vi "ADC SNR_new_beforeChn.vi"(8 "error in (no error)":errorcluster, 9 "Sequence parameters":string[][](array[string])=[["Min limit", "Max limit", "Register sheet file", "Register Sheet"], ["", "", "CC2600.xls", "TX_BLE;Trim"], ["Reg write (addr;value)", "Operating frequency [Hz]", "", ""], ["NA", "2.44G", "", ""]], 10 "Run type":i32, 11 "Method parameters":T4={"Dev"={"Do not disturb DUT"=FALSE, "XOSC"=32000000.0, "Board type"="", "EM"="", "Configure tempboard"=TRUE, "Device specific info"=[], "Generic Object"=refnum}, "Method"={"Run type"=1, "Test name"="Current LPM2 4", "Comment"="", "Results folder"="", "AFC"=enum."Off", "Method name"="Current LPM2 4", "Method results"={"Excel brief report"=FALSE, "Spotfire report"=FALSE, "Starfish report"=FALSE}, "Operator"="", "Reference time"=timestamp(0 s since 1904-01-01), "AFC delay"=0.0, "Initialization"=enum."Enabled", "MD5 Sum"="", "HW addon board"=enum."None", "AFC Regsheet"="", "AFC Regfile"=path "", "dummy"=0.0}, "Inst"={"Instr"={"PS1"={"Name"="", "GPIB address"="", "VISA session"=""}, "PS2"={"Name"="", "GPIB address"="", "VISA session"=""}, "TC1"={"Name"="", "GPIB address"="", "VISA session"=""}, "TC2"={"Name"="", "GPIB address"="", "VISA session"=""}, "SA1"={"Name"="", "GPIB address"="", "VISA session"=""}, "SA2"={"Name"="", "GPIB address"="", "VISA session"=""}, "SG1"={"Name"="", "GPIB address"="", "VISA session"=""}, "SG2"={"Name"="", "GPIB address"="", "VISA session"=""}, "SG3"={"Name"="", "GPIB address"="", "VISA session"=""}, "MI1"={"Name"="", "GPIB address"="", "VISA session"=""}, "MI2"={"Name"="", "GPIB address"="", "VISA session"=""}, "SW SA"={"Name"="", "Controller addr"=""}, "SW SG"={"Name"="", "Controller addr"=""}, "MI3"={"Name"="", "GPIB address"="", "VISA session"=""}}, "Switchbox"={"RF Path"=0, "Cal compensation"=enum."TX", "Switchbox gain mode"="", "State"=enum."TX"}, "Instr to control (i.e. SA1)"="Default", "Intrument info string"=""}, "Sequence parameters"=[["Weight", "Min Limit", "Max Limit", "Register Sheet", "", "", "", "", "", "", "", "", ""], ["Vital", "", "1", "LPM2", "", "", "", "", "", "", "", "", ""], ["Resolution", "Reg write (addr;value)", "Chip mode", "Range", "", "", "", "", "", "", "", "", ""], ["u", "NA", "", "auto", "", "", "", "", "", "", "", "", ""]], "Cond"={"Temp logged"=25.0, "VDD1_PS1_6V"=-999.0, "VDD2_PS1_25V"=-999.0, "VDD4_PS2_25V"=-999.0, "VDD3_PS2_6V"=-999.0}, "Meas config"={"X-axis inner loop index"=32000000, "Y-axis outer loop index"=32000000, "X-axis"=[], "Y-axis"=[], "X-axis array req size"=32000000, "Y-axis array req size"=32000000, "Param description"=[], "Use meas clust for reporting"=FALSE, "Parameter index (page)"=0, "X-axis name"="", "Y-axis name"=""}} {"Cond"."VDD3_PS2_6V" format="%.3f"; "Cond"."VDD4_PS2_25V" format="%.3f"; "Cond"."VDD2_PS1_25V" format="%.3f"; "Cond"."VDD1_PS1_6V" format="%.3f"; "Method"."dummy" format="%.1p"; "Method"."AFC delay" format="%.1p"; "Dev"."XOSC" format="%.3p"}) -> (0 "error out":errorcluster, 1 "End method error":T2, 2 "Short Results":string[](array[string])=["0.00", "0.00", "0.00", "0.00"], 3 "Result summary":string[][](array[string])=[["Critical", "Output Power@2405 MHz", "-3", "4", "dBm"], ["Critical", "Output Power@2410 MHz", "-3", "4", "dBm"]])   [LabVIEW 2019]
doc: "[AutoDocStart]Performs crystal accuracy measurements. Measures the offset from ideal frequency. Primarily used for tuning XOSC capacitors and verifying XOSC trims.\n\nSweeping parameters: operating frequency, OSC override value and VDDR level\n\nResults: Offset frequency in ppm[AutoDocEnd]"
uses:
  User Lib/Utilities/Cluster definitions/Method input.ctl
  User Lib/Utilities/Cluster definitions/Device specific info.ctl
  User Lib/Utilities/Controls/Automatic Frequency Compensation types.ctl
  User Lib/Utilities/Controls/Method Reports.ctl
  User Lib/Utilities/Cluster definitions/Method Initialization.ctl
  User Lib/Utilities/Controls/HW addon boards.ctl
  User Lib/Utilities/Cluster definitions/Instr clust.ctl
  User Lib/Utilities/Switchbox control/SwitchBox_State._ENUMctl.ctl
  User Lib/Utilities/Cluster definitions/End method error cluster.ctl
  User Lib/Utilities/Cluster definitions/DUT vdd control.ctl
  User Lib/Utilities/Cluster definitions/DUT VDD4.ctl
  User Lib/Utilities/Cluster definitions/DUT VDD3.ctl
  User Lib/Utilities/Cluster definitions/DUT VDD2.ctl
  User Lib/Utilities/Cluster definitions/DUT VDD1.ctl
  User Lib/Generic chip methods/Classes/Generic_EM/Chameleon/Loki/Loki.lvclass
  <vilib>/Utility/error.llb/Clear Errors.vi
  User Lib/Generic chip methods/Classes/Generic_EM/Chameleon/65nm.lvclass
  C:/Kharon/User Lib/Generic chip methods/Classes/Generic_EM/Generic_EM/Generic_EM.lvclass
  User Lib/Generic chip methods/board_to_chip_type.vi
  User Lib/Generic chip methods/Classes/Get_Class_init.vi
  User Lib/Generic chip methods/Classes/Generic_EM/Generic_EM/Generic_EM.lvclass
panel:
  in  "Tab Control":T1(tab)
  out "Dynamic Parameters":T3={"SNR"=nan, "SNRD"=nan, "THD"=nan, "ENOB (SNRD)"=nan, "SFDR"=nan, "ENOB (SNR)"=nan, "Noise Power"=nan, "Signal power"=nan} {"Signal power" format="%.6f"; "Noise Power" format="%.2f"; "ENOB (SNR)" format="%.2f"; "SFDR" format="%.2f"; "ENOB (SNRD)" format="%.2f"; "THD" format="%.2f"; "SNRD" format="%.2f"; "SNR" format="%.2f"}
  out "ADC samples":u32[](array[numeric])
  out "Output Response [All DUTs]":u32[][](array[numeric])
  out "SNR":dbl
  out "Noise Power":dbl
  out "Signal power":dbl
  out "ENOB (SNR)":dbl
  out "detected Throughput":dbl=200065.4236150998
  # "°C"
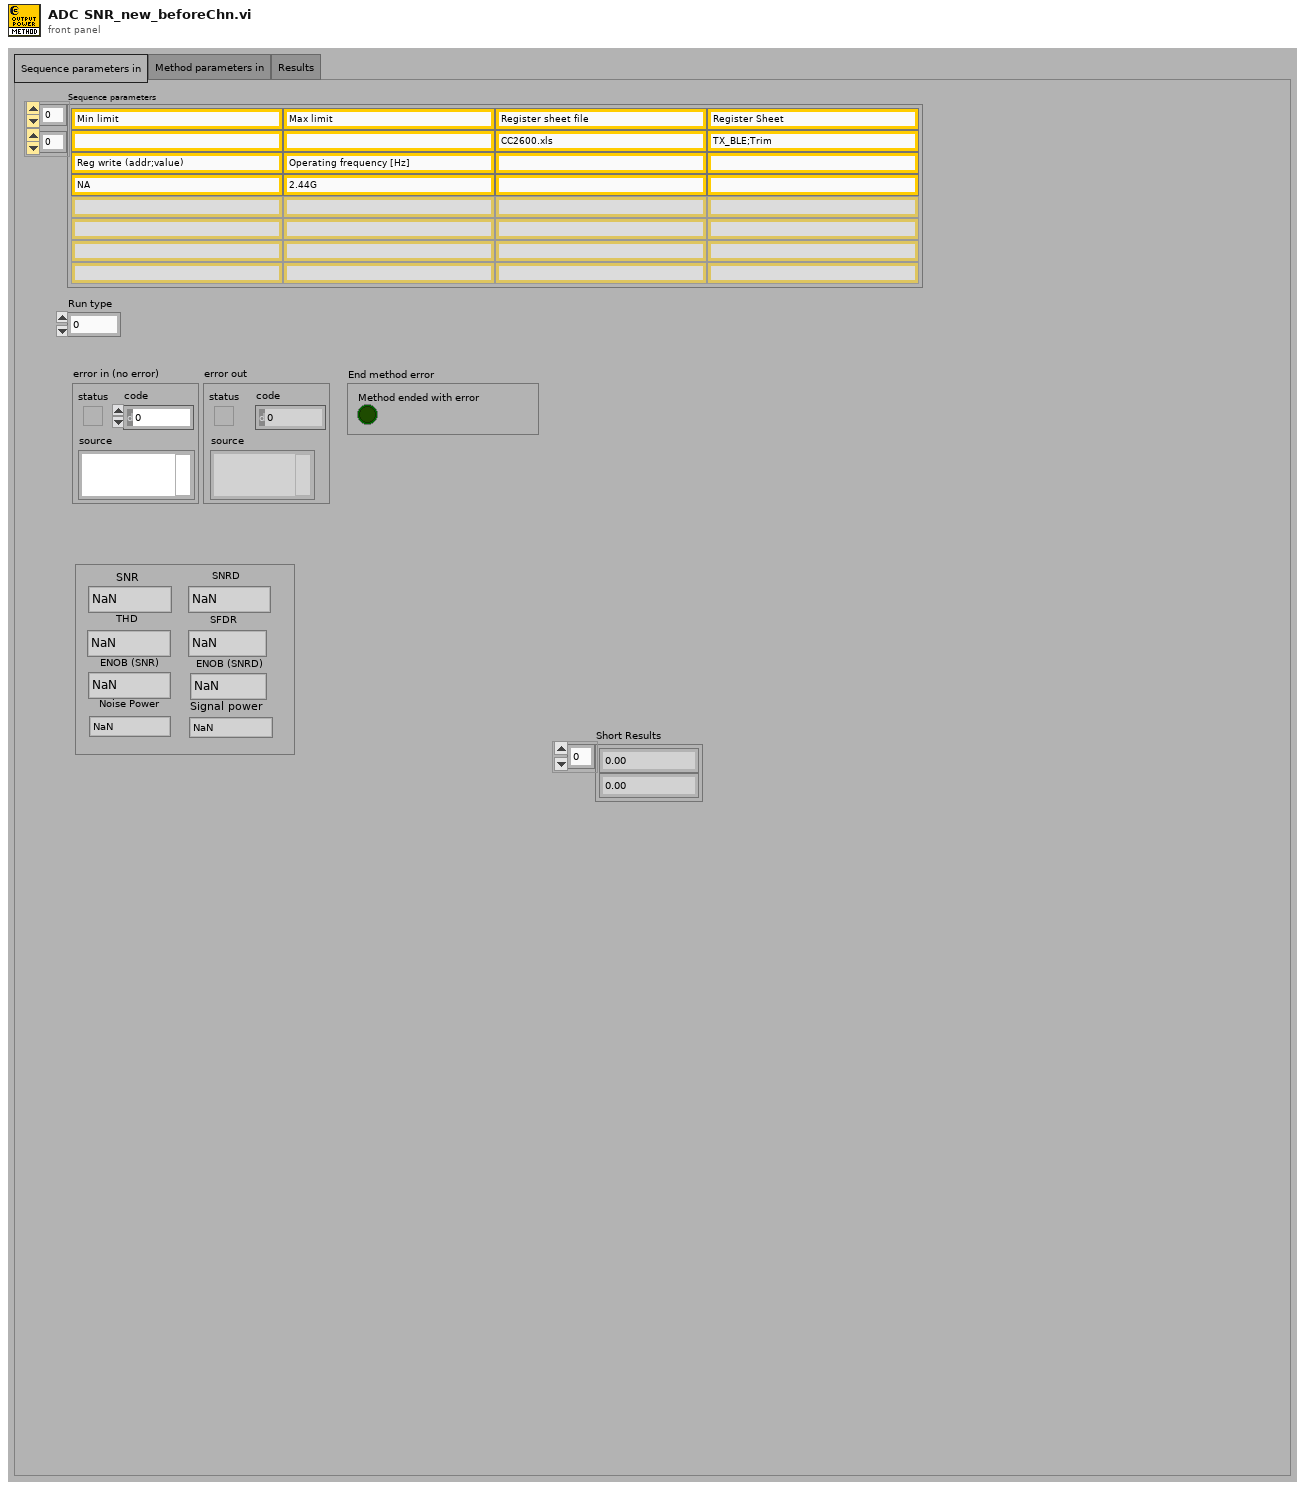
[diagram p1: front panel]
types:
  T1 = enum32{"Sequence parameters in", "Method parameters in", "Results"}
  T2 = typedef "End method error cluster.ctl" = cluster{"Method ended with error":bool}
  T3 = cluster{"SNR":dbl, "SNRD":dbl, "THD":dbl, "ENOB (SNRD)":dbl, "SFDR":dbl, "ENOB (SNR)":dbl, "Noise Power":dbl, "Signal power":dbl}
  T4 = typedef "Method input.ctl" = cluster{"Dev":cluster{"Do not disturb DUT":bool, "XOSC":dbl, "Board type":string, "EM":string, "Configure tempboard":bool, "Device specific info":T5[], "Generic Object":refnum<class>}, "Method":cluster{"Run type":i32, "Test name":string, "Comment":string, "Results folder":string, "AFC":T6, "Method name":string, "Method results":T7, "Operator":string, "Reference time":timestamp, "AFC delay":dbl, "Initialization":T8, "MD5 Sum":string, "HW addon board":T9, "AFC Regsheet":string, "AFC Regfile":path, "dummy":dbl}, "Inst":T10, "Sequence parameters":string[][], "Cond":cluster{"Temp logged":dbl, "VDD1_PS1_6V":dbl, "VDD2_PS1_25V":dbl, "VDD4_PS2_25V":dbl, "VDD3_PS2_6V":dbl}, "Meas config":cluster{"X-axis inner loop index":i32, "Y-axis outer loop index":i32, "X-axis":string[], "Y-axis":string[], "X-axis array req size":i32, "Y-axis array req size":i32, "Param description":string[][], "Use meas clust for reporting":bool, "Parameter index (page)":i32, "X-axis name":string, "Y-axis name":string}}
  T5 = typedef "Device specific info.ctl" = cluster{"EM number":u8, "IP address":string, "Enabled":bool, "Slot no":u8, "RF path":u8, "EM name":string, "Wafer info":string, "AFC frequency ppm":dbl, "Register writes":string[][], "Meas data":string[][][], "Device comment":string}
  T6 = typedef "Automatic Frequency Compensation types.ctl" = enum16{"Off", "Compensate Instrument frequency", "Compensate DUT frequency", "Predictive - Compensate Instrument frequency", "Predictive - Compensate DUT frequency", "Do not skip re-init - Compensate Instrument frequency", "Do not skip re-init - Compensate DUT frequency"}
  T7 = typedef "Method Reports.ctl" = cluster{"Excel brief report":bool, "Spotfire report":bool, "Starfish report":bool}
  T8 = typedef "Method Initialization.ctl" = enum16{"Enabled", "Skip Instr and Device Init", "Enabled with Separate Flash", "Set PS, Device Init and Skip Instr Init", "Skip Device Init"}
  T9 = typedef "HW addon boards.ctl" = enum16{"None", "Current meas 5EM", "Stresstest 10EM"}
  T10 = typedef "Instr clust.ctl" = cluster{"Instr":cluster{"PS1":cluster{"Name":string, "GPIB address":string, "VISA session":refnum<visa-resource-name>}, "PS2":cluster{"Name":string, "GPIB address":string, "VISA session":refnum<visa-resource-name>}, "TC1":cluster{"Name":string, "GPIB address":string, "VISA session":refnum<visa-resource-name>}, "TC2":cluster{"Name":string, "GPIB address":string, "VISA session":refnum<visa-resource-name>}, "SA1":cluster{"Name":string, "GPIB address":string, "VISA session":refnum<visa-resource-name>}, "SA2":cluster{"Name":string, "GPIB address":string, "VISA session":refnum<visa-resource-name>}, "SG1":cluster{"Name":string, "GPIB address":string, "VISA session":refnum<visa-resource-name>}, "SG2":cluster{"Name":string, "GPIB address":string, "VISA session":refnum<visa-resource-name>}, "SG3":cluster{"Name":string, "GPIB address":string, "VISA session":refnum<visa-resource-name>}, "MI1":cluster{"Name":string, "GPIB address":string, "VISA session":refnum<visa-resource-name>}, "MI2":cluster{"Name":string, "GPIB address":string, "VISA session":refnum<visa-resource-name>}, "SW SA":cluster{"Name":string, "Controller addr":string}, "SW SG":cluster{"Name":string, "Controller addr":string}, "MI3":cluster{"Name":string, "GPIB address":string, "VISA session":refnum<visa-resource-name>}}, "Switchbox":cluster{"RF Path":i32, "Cal compensation":enum16{"TX", "RX", "Interferer", "No compensation", "Interferer2"}, "Switchbox gain mode":string, "State":T11}, "Instr to control (i.e. SA1)":string, "Intrument info string":string}
  T11 = typedef "SwitchBox_State._ENUMctl.ctl" = enum16{"TX", "RX", "SP:TX", "SP:RX", "SW:TX", "SW:RX"}
  T12 = cluster{"Path to Save plot":path, "Path to Raw Data plot":path}
  T13 = cluster{"Fundamental Frequency":dbl, "Sampling Frequncy":dbl, "No of Harmonics":u8, "Window":enum16{"None ", "Hanning", "Hamming", "Blackman-Harris", "Exact Blackman", "Blackman", "Flat Top", "4 Term B-Harris ", "7 Term B-Harris"}, "Blackman (fundamental power) bins)":dbl}
  T14 = cluster{"Save INL/DNL Plot(Ramp)":bool, "Save SNR Plot":bool, "Save INL/DNL Plot(Sine)":bool, "Save INL/DNL Raw Data(Ramp)":bool, "Save SNR Raw Data":bool, "Save INL/DNL Raw Data(Sine)":bool, "Save DC Raw data":bool, "Save  Raw Data(Sine)":bool}
  T15 = typedef "DUT vdd control.ctl" = cluster{"VDD4 config":T16, "VDD3 config":T17, "VDD2 config":T18, "VDD1 config":T19}
  T16 = typedef "DUT VDD4.ctl" = u16
  T17 = typedef "DUT VDD3.ctl" = u16
  T18 = typedef "DUT VDD2.ctl" = u16
  T19 = typedef "DUT VDD1.ctl" = u16
  T20 = enum32{"NI Card Settings", "Memory Read Setting", "DC Capture", "ADC Ramp", "ADC Sine", "SNR", "Cap Calibration"}
  T21 = enum32{"Read from Memory", "Read .dat file", "NI Card Capture", "None"}
  T22 = typedef "TFW ResponseData.ctl" = cluster{"errorCode":u32, "executionTime":u32, "processedCmdWord":u32, "responsePar":u32[], "actionCode":u32, "cmdStatus":u16}
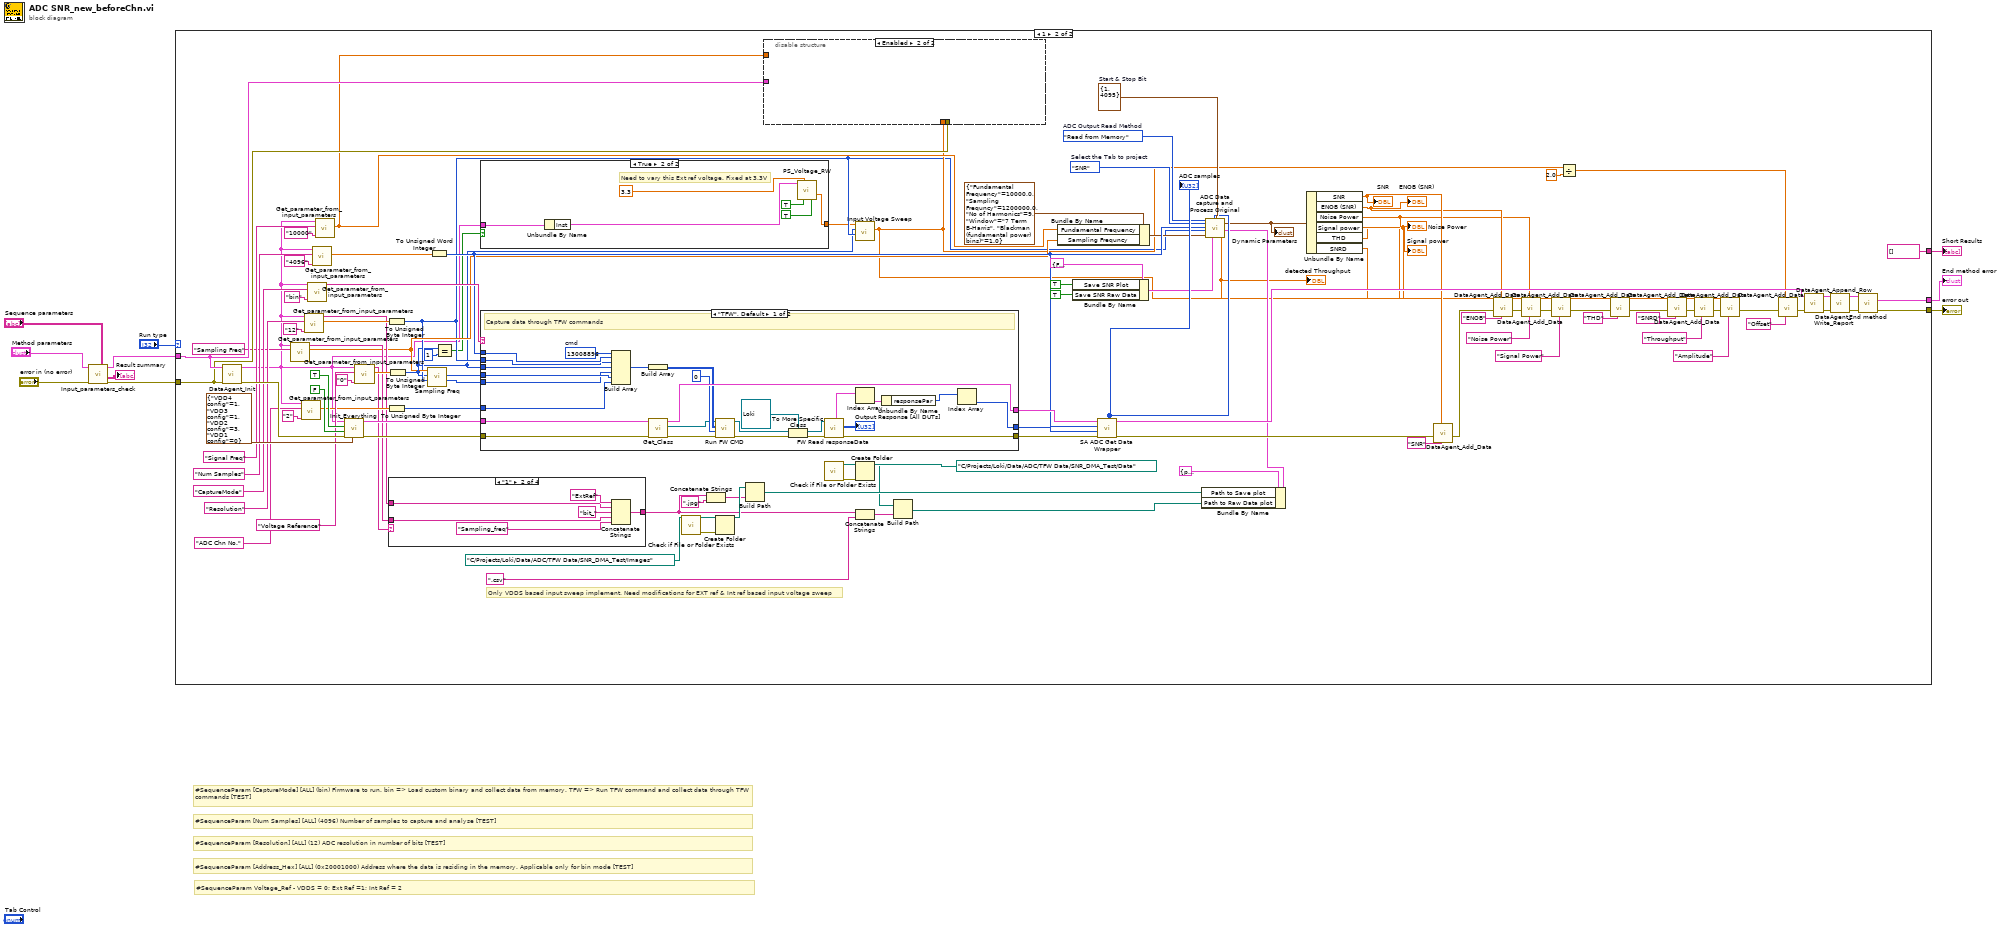
[diagram p0: block diagram]
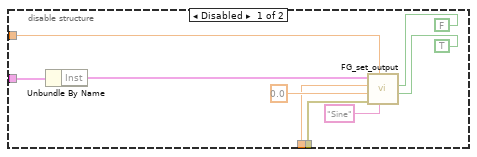
[diagram p3: hidden frame]
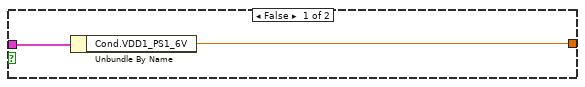
[diagram p4: hidden frame]
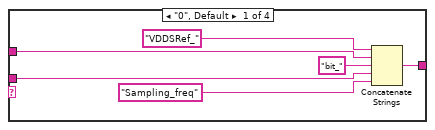
[diagram p5: hidden frame]
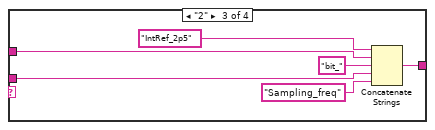
[diagram p6: hidden frame]
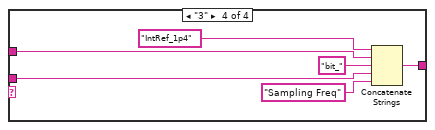
[diagram p7: hidden frame]
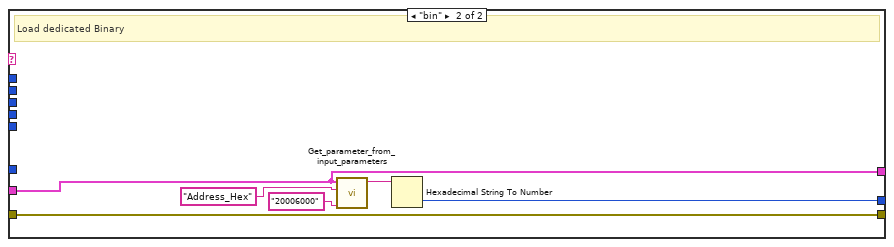
[diagram p8: hidden frame]
diagram:
  # "#SequenceParam Voltage_Ref - VDDS = 0; Ext Ref =1; Int Ref = 2"
  # "#SequenceParam [Num Samples] [ALL] (4096) Number of samples to capture and analyse [TEST]"
  # "#SequenceParam [CaptureMode] [ALL] (bin) Firmware to run. bin => Load custom binary and collect data from memory. TFW => Run TFW command and collect data through TFW commands [TEST]"
  # "#SequenceParam [Address_Hex] [ALL] (0x20001000) Address where the data is residing in the memory. Applicable only for bin mode [TEST]"
  # "#SequenceParam [Resolution] [ALL] (12) ADC resolution in number of bits [TEST]"
  n1 = call "Input_parameters_check.vi"("Sequence parameters"="Sequence parameters", "error in"="error in (no error)", "Method cluster in"="Method parameters") -> ("error out"=w9:errorcluster, "Result summary"=→"Result summary":string[][], "Method cluster out"=w5:T4)  [unwired: 6 in]
  n2 = case shown="1" "Run type" {
    tunnel: w9 -> [w11 w36]
    tunnel: [w11 w120] -> w10
    tunnel: w5 -> [_ w37]
    tunnel: [_ w119] -> w4
    tunnel: [_ string[] []] -> w1
    frame 0, Default {
      # "Run type 0 is only for formatting the result summary"
    }
    frame 1 {
      w46 = cluster{"Start":i32, "Stop":i32} {"Start"=1, "Stop"=4095}  # Start & Stop Bit
      w39 = T20."SNR"  # Select the Tab to project
      w40 = T21."Read from Memory"  # ADC Output Read Method
      # "Only VDDS based input sweep implement. Need modifications for EXT ref & Int ref based input voltage sweep"
      n3 = call "DataAgent_Init.vi"("error in (no error)"=w36, "Method cluster in"=w37) -> ("error out"=w117:errorcluster, "Method cluster out"=w13:T4)  [unwired: 8 in]
      n4 = call "Get_parameter_from_input_parameters.vi"("Parameter name"="Sampling Freq", "Method cluster (if input param empty)"=w13) -> ("value as DBL"=w23:dbl, "value as String"=w30:string)  [unwired: 3 in, 5 out]
      n5 = call "Get_parameter_from_input_parameters.vi"("Default value (used if not specified on Front Panel)"="2", "Parameter name"="ADC Chn No.", "Method cluster (if input param empty)"=w13) -> ("value as DBL"=w52:dbl)  [unwired: 2 in, 6 out]
      n6 = call "Get_parameter_from_input_parameters.vi"("Default value (used if not specified on Front Panel)"="12", "Parameter name"="Resolution" ("SA_ param name"), "Method cluster (if input param empty)"=w13) -> ("value as DBL"=w49:dbl, "value as String"=w48:string)  [unwired: 2 in, 5 out]
      n7 = call "Get_parameter_from_input_parameters.vi"("Default value (used if not specified on Front Panel)"="bin", "Parameter name"="CaptureMode" ("SA_ param name"), "Method cluster (if input param empty)"=w13) -> ("value as String"=w108:string)  [unwired: 2 in, 6 out]
      n8 = call "Get_parameter_from_input_parameters.vi"("Default value (used if not specified on Front Panel)"="4096", "Parameter name"="Num Samples" ("SA_ param name"), "Method cluster (if input param empty)"=w13) -> ("value as DBL"=w101:dbl)  [unwired: 2 in, 6 out]
      n9 = call "Get_parameter_from_input_parameters.vi"("Default value (used if not specified on Front Panel)"="10000", "Parameter name"="Signal Freq", "Method cluster (if input param empty)"=w13) -> ("value as DBL"=w22:dbl)  [unwired: 2 in, 6 out]
      n10 = call "Init_Everything.vi"("VDD config"=T15 {"VDD4 config"=1, "VDD3 config"=1, "VDD2 config"=3, "VDD1 config"=0}, "error in"=w117, "Support current measurement?"=FALSE, "Override VDD Config"=TRUE, "Method cluster In"=w13) -> ("error out"=w114:errorcluster, "Method cluster out"=w113:T4)  [unwired: 3 in, 2 out]
      n11 = call "Get_parameter_from_input_parameters.vi"("Default value (used if not specified on Front Panel)"="0", "Parameter name"="Voltage Reference", "Method cluster (if input param empty)"=w13) -> ("value as DBL"=w88:dbl, "value as String"=w47:string)  [unwired: 2 in, 5 out]
      n12 = To Unsigned Byte Integer(number=w49) -> (unsigned 8bit integer=w17:u8)
      n13 = To Unsigned Byte Integer(number=w52) -> (unsigned 8bit integer=w51:u8)
      n14 = To Unsigned Byte Integer(number=w88) -> (unsigned 8bit integer=w14:u8)
      n15 = case shown="\"1\"" w47 {
        tunnel: [w141 w147 w153 w156] -> w57
        tunnel: w48 -> [w139 w146 w151 w158]
        tunnel: w30 -> [w138 w145 w150 w157]
        frame "0", Default {
          n16 = Concatenate Strings("VDDSRef_" ("string"), w139, "bit_" ("string"), w138, "Sampling_freq" ("string")) -> (w141:string)
        }
        frame "1" {
          n17 = Concatenate Strings("ExtRef" ("string"), w146, "bit_" ("string"), w145, "Sampling_freq" ("string")) -> (w147:string)
        }
        frame "2" {
          n18 = Concatenate Strings("IntRef_2p5" ("string"), w151, "bit_" ("string"), w150, "Sampling_freq" ("string")) -> (w153:string)
        }
        frame "3" {
          n19 = Concatenate Strings("IntRef_1p4" ("string"), w158, "bit_" ("string"), w157, "Sampling Freq" ("string")) -> (w156:string)
        }
      }
      n20 = call "Sampling Freq.vi"("Resolution"=w17, "Voltage Ref"=w14, "Sampling Freq"=w23) -> ("LGPT Count"=w29:u16, "SCOMP"=w28:u16)  [unwired: 7 in]
      n21 = To Unsigned Word Integer(number=w101) -> (unsigned 16bit integer=w38:u16)
      n22 = Equal?(x=w14, y=u8 1) -> (x = y?=w16:bool)
      n23 = case shown="True" w16 {
        tunnel: w13 -> [w131 w137]
        tunnel: [w130 w132] -> w12
        frame False {
          n24 = Unbundle By Name(w131) -> ("Cond.VDD1_PS1_6V"=w130:dbl)
        }
        frame True {
          # "Need to vary this Ext ref voltage. Fixed at 3.3V"
          n25 = Unbundle By Name(w137) -> ("Inst"=w136:T10)
          n26 = call "PS_Voltage_RW.vi"("InstrCluster in"=w136, "Set Voltage"=3.3, "Off (F)                         On (T)"=TRUE, "Read (F)                      Write (T)"=TRUE) -> ("Output Voltage"=w132:dbl)  [unwired: 9 in, 2 out]
        }
      }
      n27 = case shown="\"TFW\", Default" w108 {
        tunnel: [w187 w188] -> w104
        tunnel: [w180 w193] -> w103
        tunnel: w114 -> [w179 w193]
        tunnel: w113 -> [w186 w188]
        tunnel: [w167 w189] -> w102
        tunnel: w38 -> [w183 _]
        tunnel: w17 -> [w166 _]
        tunnel: w28 -> [w165 _]
        tunnel: w51 -> [w164 _]
        tunnel: w14 -> [w163 _]
        tunnel: w29 -> [w162 _]
        frame "TFW", Default {
          w184 = u32 13008896  # cmd
          # "Capture data through TFW commands"
          n28 = Build Array(w184, w183, w166, w163, w162, w165, w164) -> (w182:u32[])
          n29 = Build Array(w182) -> (w181:u32[][])
          n30 = call "Get_Class.vi"("error in (no error)"=w179, "Method cluster in"=w186) -> ("error out"=w177:errorcluster, "Class Out"=w176:refnum<class "Generic_EM.lvclass">, "Method cluster out"=w187:T4)  [unwired: 6 in, 1 out]
          n31 = call-dynamic "Run FW CMD.vi"("error in (no error)"=w177, "Handler"=u8 0, "cmdBuf"=w181, "Generic_EM in"=w176) -> ("error out"=w172:errorcluster, "Generic_EM out"=w175:refnum<class "Generic_EM.lvclass">)  [unwired: 6 in]
          n32 = To More Specific Class(target class=refnum<class "Loki.lvclass"> refnum ("Loki in"), reference=w175, error in=w172) -> (specific class reference=w173:refnum<class "Loki.lvclass">, error out=w171:errorcluster)
          n33 = call "FW Read responseData.vi"("error in (no error)"=w171, "Loki in"=w173) -> ("error out"=w180:errorcluster, "Output Response [All DUTs]"=→"Output Response [All DUTs]":u32[][], "Response"=w169:T22[])  [unwired: 6 in, 1 out]
          n34 = Index Array(array=w169) -> (element=w170:T22)  [unwired: 1 in]
          n35 = Unbundle By Name(w170) -> ("responsePar"=w168:u32[])
          n36 = Index Array(array=w168) -> (element=w167:u32)  [unwired: 1 in]
        }
        frame "bin" {
          # "Load dedicated Binary"
          n37 = call "Get_parameter_from_input_parameters.vi"("Default value (used if not specified on Front Panel)"="20006000", "Parameter name"="Address_Hex" ("SA_ param name"), "Method cluster (if input param empty)"=w188) -> ("value as String"=w192:string)  [unwired: 2 in, 6 out]
          n38 = Hexadecimal String To Number(string=w192) -> (number=w189:u32)  [unwired: 2 in, 1 out]
        }
      }
      n39 = call <vilib>:"Check if File or Folder Exists.vi"("path"=path "C:/Projects/Loki/Data/ADC/TFW Data/SNR_DMA_Test/Images" ("base path")) -> ("error out"=w70:errorcluster, "dup path"=w69:path)  [unwired: 8 in, 1 out]
      n40 = Concatenate Strings(w57, ".jpg" ("string")) -> (w55:string)
      n41 = Create Folder(path (use dialog)=w69, error in=w70) -> (created path=w67:path)  [unwired: 1 in, 2 out]
      n42 = Build Path(base path=w67, name or relative path=w55) -> (appended path=w66:path)
      n43 = call <vilib>:"Check if File or Folder Exists.vi"("path"=path "C:/Projects/Loki/Data/ADC/TFW Data/SNR_DMA_Test/Data" ("base path")) -> ("error out"=w65:errorcluster, "dup path"=w64:path)  [unwired: 8 in, 1 out]
      n44 = call "Input Voltage Sweep.vi"("Resolution"=w17, "Voltage Ref"=w14, "VDDS"=w12) -> ("High Voltage"=w18:dbl)  [unwired: 8 in]
      n45 = disable-structure shown="Enabled" {
        disable-tunnel: w37 -> [w129 _]
        disable-tunnel: w36 -> [w123 _]
        disable-tunnel: w22 -> [w122 _]
        disable-tunnel: w18 -> [w121 _]
        frame Disabled {
          n46 = Unbundle By Name(w129) -> ("Inst"=w128:T10)
          n47 = call "FG_set_output.vi"("High impedance (T)"=TRUE, "Invert output"=FALSE, "Function (DC, Sine, Square, Triangle, Ramp up, Ramp down, Pulse)"="Sine", "Frequency [Hz]"=w122, "error in"=w123, "Low voltage"=0.0, "High voltage (or DC)"=w121, "InstrCluster in"=w128) -> ()  [unwired: 2 in, 2 out]
        }
        frame Enabled {
        }
      }
      n48 = Create Folder(path (use dialog)=w64, error in=w65) -> (created path=w62:path)  [unwired: 1 in, 2 out]
      n49 = Concatenate Strings(w57, ".csv" ("string")) -> (w54:string)
      n50 = Build Path(base path=w62, name or relative path=w54) -> (appended path=w61:path)
      n51 = Bundle By Name(cluster=T13 {"Fundamental Frequency"=10000.0, "Sampling Frequncy"=1200000.0, "No of Harmonics"=9, "Window"=enum."7 Term B-Harris", "Blackman (fundamental power) bins)"=1.0} ("Inputs for Dyanmic para"), "Fundamental Frequency"=w22, "Sampling Frequncy"=w23) -> (w32:T13)
      n52 = Bundle By Name(cluster=T14 {"Save INL/DNL Plot(Ramp)"=FALSE, "Save SNR Plot"=FALSE, "Save INL/DNL Plot(Sine)"=FALSE, "Save INL/DNL Raw Data(Ramp)"=FALSE, "Save SNR Raw Data"=FALSE, "Save INL/DNL Raw Data(Sine)"=FALSE, "Save DC Raw data"=FALSE, "Save  Raw Data(Sine)"=FALSE} ("Save data"), "Save SNR Plot"=TRUE, "Save SNR Raw Data"=TRUE) -> (w44:T14)
      n53 = call "SA ADC Get Data Wrapper.vi"("error in"=w103, "Data Address"=w102, "Num Samples"=w38, "Method cluster in"=w104) -> ("error out"=w106:errorcluster, "output cluster"=w105:T4, "ADC samples"=w45:u32[])  [unwired: 2 in, 3 out]
      "ADC samples" <- w45
      n54 = Bundle By Name(cluster=T12 {"Path to Save plot"=path "C:/Projects/Loki/Data/ADC/TFW Data/test.jpg", "Path to Raw Data plot"=path "C:/Projects/Loki/Data/ADC/TFW Data/test.csv"} ("path to save"), "Path to Save plot"=w66, "Path to Raw Data plot"=w61) -> (w42:T12)
      n55 = call "ADC Data capture and Process Original.vi"("ADC Output Read Method"=w40, "Select the Tab to project"=w39, "No.of samples(SNR)"=w38, "Resolution"=w17, "Inputs for Dyanmic para"=w32, "Save data"=w44, "Waveform"=w45, "Start & Stop Bit"=w46, "path to save"=w42) -> ("detected Throughput"=w41:dbl, "Dynamic Parameters"=w43:T3)  [unwired: 12 in, 5 out]
      "Dynamic Parameters" <- w43
      "detected Throughput" <- w41
      n56 = Unbundle By Name(w43) -> ("SNR"=w91:dbl, "ENOB (SNR)"=w90:dbl, "Noise Power"=w76:dbl, "Signal power"=w75:dbl, "THD"=w74:dbl, "SNRD"=w73:dbl)
      "SNR" <- w91
      "Noise Power" <- w76
      "Signal power" <- w75
      "ENOB (SNR)" <- w90
      n57 = call "DataAgent_Add_Data.vi"("ColumnName"="SNR" ("Default Value"), "Data"=w91, "error in (no error)"=w106) -> ("error out"=w95:errorcluster)  [unwired: 8 in]
      n58 = call "DataAgent_Add_Data.vi"("ColumnName"="ENOB" ("Default Value"), "Data"=w90, "error in (no error)"=w95) -> ("error out"=w84:errorcluster)  [unwired: 8 in]
      n59 = call "DataAgent_Add_Data.vi"("ColumnName"="Noise Power", "Data"=w76, "error in (no error)"=w84) -> ("error out"=w83:errorcluster)  [unwired: 8 in]
      n60 = call "DataAgent_Add_Data.vi"("ColumnName"="Signal Power", "Data"=w75, "error in (no error)"=w83) -> ("error out"=w78:errorcluster)  [unwired: 8 in]
      n61 = Divide(x=w18, y=2.0) -> (x/y=w21:dbl)
      n62 = call "DataAgent_Add_Data.vi"("ColumnName"="THD", "Data"=w74, "error in (no error)"=w78) -> ("error out"=w77:errorcluster)  [unwired: 8 in]
      n63 = call "DataAgent_Add_Data.vi"("ColumnName"="SNRD", "Data"=w73, "error in (no error)"=w77) -> ("error out"=w72:errorcluster)  [unwired: 8 in]
      n64 = call "DataAgent_Add_Data.vi"("ColumnName"="Throughput", "Data"=w41, "error in (no error)"=w72) -> ("error out"=w19:errorcluster)  [unwired: 8 in]
      n65 = call "DataAgent_Add_Data.vi"("ColumnName"="Amplitude", "Data"=w18, "error in (no error)"=w19) -> ("error out"=w24:errorcluster)  [unwired: 8 in]
      n66 = call "DataAgent_Add_Data.vi"("ColumnName"="Offset", "Data"=w21, "error in (no error)"=w24) -> ("error out"=w25:errorcluster)  [unwired: 8 in]
      n67 = call "DataAgent_Append_Row.vi"("error in (no error)"=w25, "Method cluster in"=w105) -> ("error out"=w97:errorcluster, "Method cluster out"=w98:T4)  [unwired: 8 in]
      n68 = call "DataAgent_Write_Report.vi"("error in (no error)"=w97, "Method cluster in"=w98) -> ("error out"=w116:errorcluster, "Method cluster out"=w115:T4)  [unwired: 8 in]
      n69 = call "End method.vi"("error in"=w116, "Method cluster in"=w115) -> ("error out"=w120:errorcluster, "End method error"=w119:T2)  [unwired: 7 in, 1 out]
    }
  }
  "error out" <- w10
  "End method error" <- w4
  "Short Results" <- w1
